vi "LabVIEW Basics #10 - Mouse and Keyboard Control.vi"() -> ()   [LabVIEW 2020]
uses:
  <vilib>/MakerHub/LINX/Public/Utilities/Open Serial.vi
  <vilib>/MakerHub/LINX/Public/Sensors/Motion/Servo/Servo Open N Channels.vi
  <vilib>/MakerHub/LINX/Public/Sensors/Motion/Servo/Servo Set Pulse Width N Channels.vi
  <vilib>/MakerHub/LINX/Public/Sensors/Motion/Servo/Servo Close N Channels.vi
  <vilib>/MakerHub/LINX/LMH-LINX.lvlib
  <vilib>/MakerHub/LINX/Public/Sensors/Motion/Servo/Servo.lvlib
panel:
  out "Mouse Control":picture
  in  "Pan Servo":u16(slide)=2200 step=100 scale=500.0..2500.0
  in  "Tilt Servo":u16(slide)=1400 step=100 scale=500.0..2500.0
  in  "Servo Channels":u8[](array[numeric])
  out "Device Name":string
  in  "Stop":bool
  # "General Controls"
  # "Servo Controls"
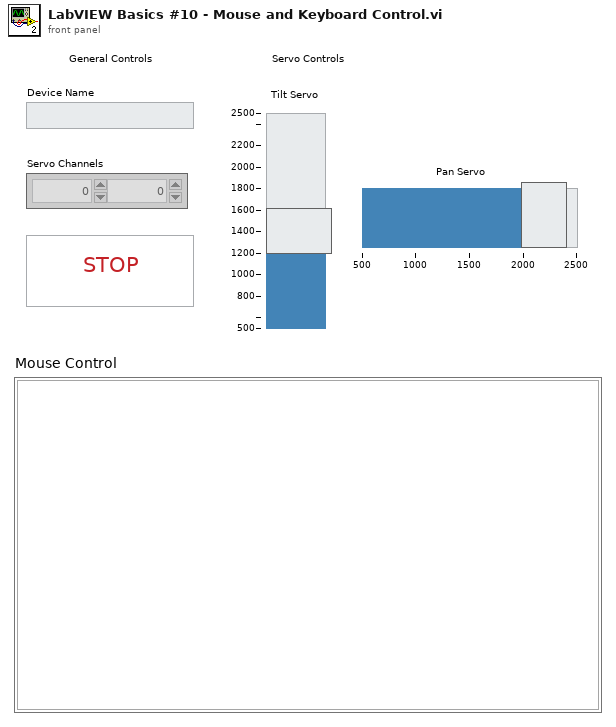
[diagram p1: front panel]
types:
  T1 = typedef "LMH-LINX.lvlib/LINX Ref.ctl" = cluster{"IO":T2, "Interface":T3, "LINX Device Config":T4}
  T2 = typedef "LMH-LINX.lvlib/Platform.ctl" = enum16{"Remote", "Local"}
  T3 = typedef "LMH-LINX.lvlib/Interface.ctl" = enum16{"Serial", "TCP"}
  T4 = typedef "LMH-LINX.lvlib/Device.lvlib/LINX Device Config.ctl" = cluster{"Interface":T3, "COM Port":refnum<visa-resource-name>, "TCP Configuration":T5, "Device Family":u8, "Device ID":u8, "Device Name":string, "TCP Ref":refnum<k5>, "Channels":T6}
  T5 = typedef "LMH-LINX.lvlib/Device.lvlib/TCP Config.ctl" = cluster{"IP Address":string, "Port":u16}
  T6 = typedef "LMH-LINX.lvlib/Channels.ctl" = cluster{"DI":u8[], "DO":u8[], "AI":u8[], "AO":u8[], "PWM":u8[], "QE":u8[], "UART":u8[], "I2C 2":u8[], "SPI":u8[], "CAN":u8[], "Servo":u8[], "AI Ref (V)":dbl, "AI Resolution (Bits)":u8, "AO Ref (V)":dbl, "AO Resolution (Bits)":u8}
  T7 = typedef "eventvkey.ctl" = enum16{"ASCII", "Enter", "Return", "Shift", "Ctrl", "Alt", "Cmd", "Opt", "Caps", "NumLock", "Clear", "Break", "Up", "Down", "Left", "Right", "Insert", "Delete", "Home", "End", "PageUp", "PageDown", "Escape", "Help", "Pause", "ScrollLock", "F1", "F2", "F3", "F4", "F5", "F6", "F7", "F8", "F9", "F10", "F11", "F12", "F13", "F14", "F15", "F16", "F17", "F18", "F19", "F20", "F21", "F22", "F23", "F24", "Play", "VolumeUp", "VolumeDown", "Mute", "Two Byte Char"}
  T8 = typedef "LVMouseTypeDef.ctl" = cluster{"Mouse Position":cluster{"X":i32, "Y":i32}, "Mouse Modifiers":cluster{"Button Down":bool, "Shift Mod":bool, "Menu Mod":bool, "Option Mod":bool}}
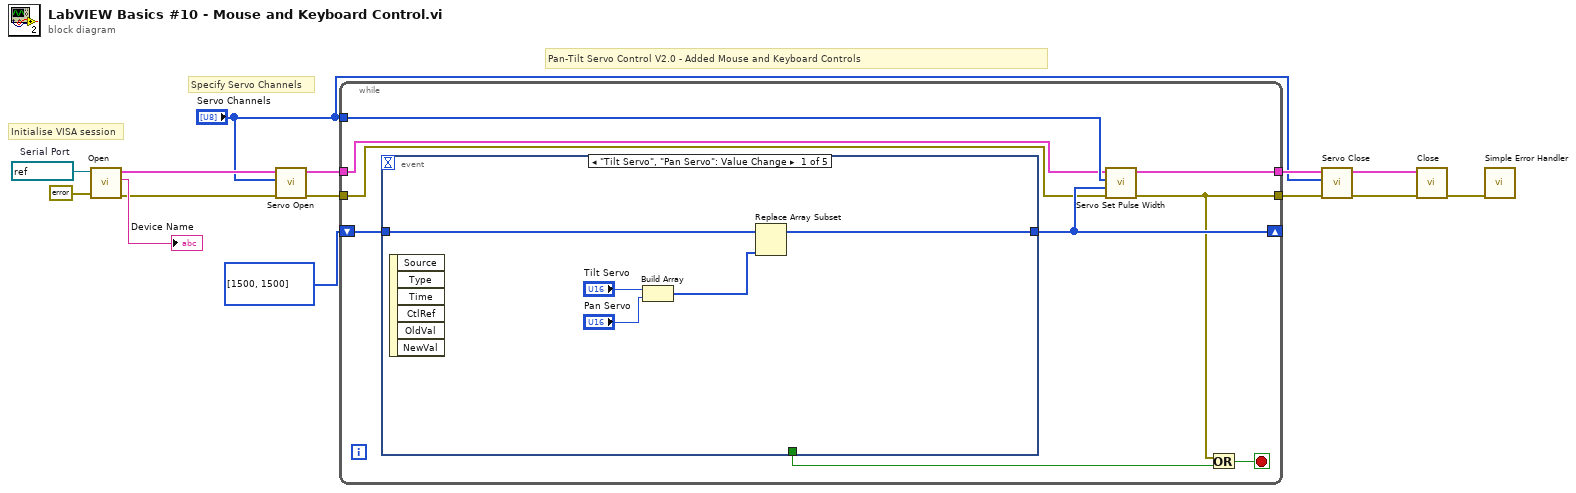
[diagram p0: block diagram]
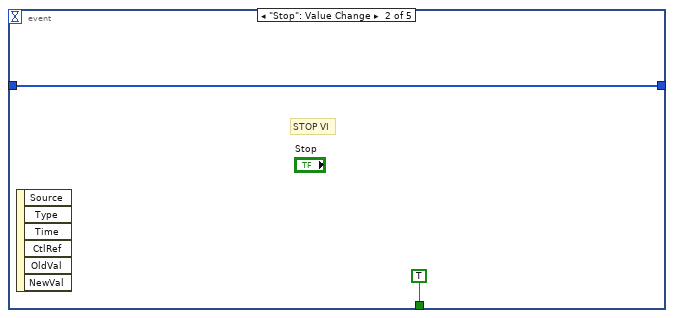
[diagram p2: hidden frame]
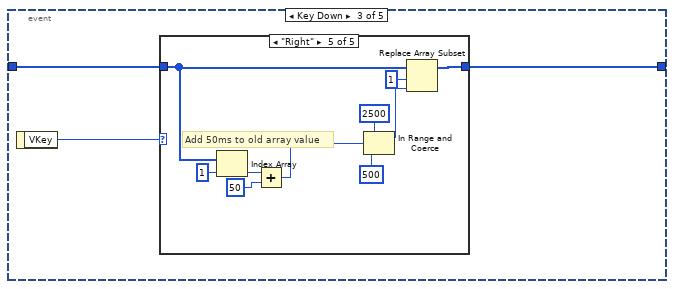
[diagram p3: hidden frame]
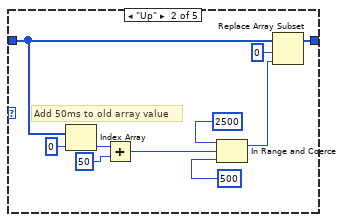
[diagram p5: hidden frame]
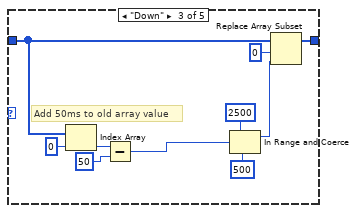
[diagram p6: hidden frame]
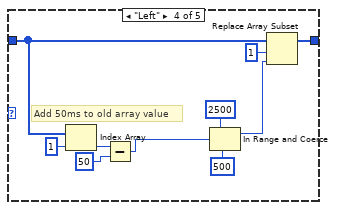
[diagram p7: hidden frame]
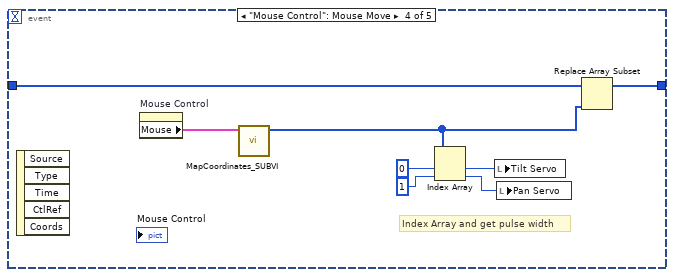
[diagram p8: hidden frame]
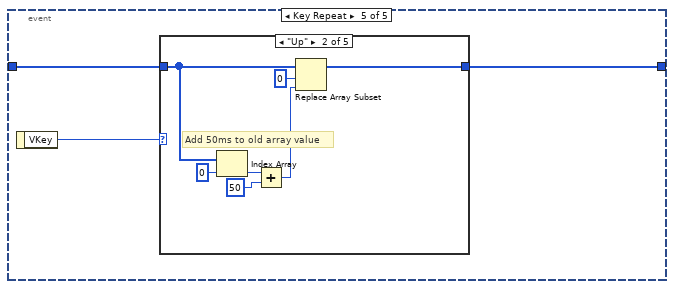
[diagram p9: hidden frame]
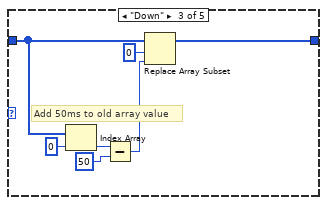
[diagram p11: hidden frame]
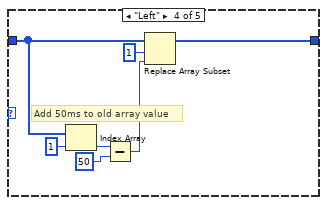
[diagram p12: hidden frame]
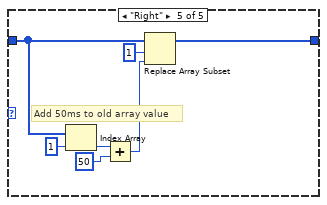
[diagram p13: hidden frame]
diagram:
  w14 = refnum<visa-resource-name> "COM5"  # Serial Port
  # "Specify Servo Channels"
  # "Initialise VISA session"
  # "Pan-Tilt Servo Control V2.0 - Added Mouse and Keyboard Controls"
  n1 = call-poly <vilib>:"Open.vi"("Error In"=errorcluster {"status"=FALSE, "code"=0, "source"=""}, "Serial Port"=w14) -> ("Error Out"=w7:errorcluster, "Device Name"=→"Device Name":string, "LINX Resource"=w6:T1)  [unwired: 7 in]
  n2 = call-poly <vilib>:"Servo Open.vi"("Error In"=w7, "Servo Channels"="Servo Channels", "LINX Resource"=w6) -> ("Error Out"=w5:errorcluster, "LINX Resource"=w8:T1)  [unwired: 7 in]
  n3 = while {
    tunnel: w8 -> [w18]
    tunnel: w5 -> [w17]
    tunnel: "Servo Channels" -> [w20]
    shift-right: [w19] -> _
    shift-left: u16[] [1500, 1500] -> [w21]
    tunnel: [w16] -> w4
    tunnel: [w15] -> w3
    stop <- w23 stop-if-true
    n4 = event shown="[0] \"Tilt Servo\", \"Pan Servo\": Value Change" {
      selector: _ -> [_ _ _ _ _]
      dyn-events: _ -> [_ _ _ _ _]
      timeout: _ -> [_ _ _ _ _]
      tunnel: [_ TRUE ("Stop") _ _ _] -> w22
      tunnel: [w25 w29 w31 w81 w83] -> w19
      tunnel: w21 -> [w26 w29 w32 w80 w84]
      event "Tilt Servo", "Pan Servo": Value Change {
        n5 = event-data() -> ()  [unwired: 1 in, 6 out]
        n6 = Build Array("Tilt Servo", "Pan Servo") -> (w24:u16[])
        n7 = Replace Array Subset(array=w26, new element=w24) -> (w25:u16[])  [unwired: 1 in]
      }
      event "Stop": Value Change {
        # "STOP VI"
        n8 = event-data() -> ()  [unwired: 1 in, 6 out]
      }
      event Key Down {
        n9 = event-data() -> ("VKey"=w33:T7)  [unwired: 1 in]
        n10 = case shown="\"Right\"" w33 {
          tunnel: w32 -> [w34 w42 w52 w62 w72]
          tunnel: [w34 w44 w54 w64 w74] -> w31
          frame "ASCII", Default {
            # "do nothing"
          }
          frame "Up" {
            # "Add 50ms to old array value"
            n11 = Index Array(array=w42, index=0) -> (element=w40:u16)
            n12 = Add(x=w40, y=u16 50) -> (x+y=w38:u16)
            n13 = In Range and Coerce(upper limit=u16 2500, x=w38, lower limit=u16 500 ("x+y")) -> (coerced(x)=w36:u16)  [unwired: 1 out]
            n14 = Replace Array Subset(array=w42, new element=w36, index=0) -> (w44:u16[])
          }
          frame "Down" {
            # "Add 50ms to old array value"
            n15 = Index Array(array=w52, index=0) -> (element=w50:u16)
            n16 = Subtract(x=w50, y=u16 50) -> (x-y=w46:u16)
            n17 = In Range and Coerce(upper limit=u16 2500, x=w46, lower limit=u16 500 ("x+y")) -> (coerced(x)=w45:u16)  [unwired: 1 out]
            n18 = Replace Array Subset(array=w52, new element=w45, index=0) -> (w54:u16[])
          }
          frame "Left" {
            # "Add 50ms to old array value"
            n19 = Index Array(array=w62, index=1) -> (element=w60:u16)
            n20 = Subtract(x=w60, y=u16 50) -> (x-y=w55:u16)
            n21 = In Range and Coerce(upper limit=u16 2500, x=w55, lower limit=u16 500 ("x+y")) -> (coerced(x)=w58:u16)  [unwired: 1 out]
            n22 = Replace Array Subset(array=w62, new element=w58, index=1) -> (w64:u16[])
          }
          frame "Right" {
            # "Add 50ms to old array value"
            n23 = Index Array(array=w72, index=1) -> (element=w70:u16)
            n24 = Add(x=w70, y=u16 50) -> (x+y=w66:u16)
            n25 = In Range and Coerce(upper limit=u16 2500, x=w66, lower limit=u16 500 ("x+y")) -> (coerced(x)=w65:u16)  [unwired: 1 out]
            n26 = Replace Array Subset(array=w72, new element=w65, index=1) -> (w74:u16[])
          }
        }
      }
      event "Mouse Control": Mouse Move {
        # "Index Array and get pulse width"
        n27 = event-data() -> ()  [unwired: 1 in, 5 out]
        n28 = property on="Mouse Control" class="Pict"() -> ("Mouse"=w82:T8)  [unwired: 2 in, 2 out]
        n29 = call "MapCoordinates_SUBVI.vi"("Mouse"=w82) -> ("Pulse Width Array"=w79:u16[])  [unwired: 10 in]
        n30 = Index Array(array=w79, index #1=0 ("index"), index #2=1 ("index")) -> (element #1=w75:u16, element #2=w76:u16)
        n31 = local write "Tilt Servo"(w75) -> ()
        n32 = local write "Pan Servo"(w76) -> ()
        n33 = Replace Array Subset(array=w80, new element=w79) -> (w81:u16[])  [unwired: 1 in]
      }
      event Key Repeat {
        n34 = event-data() -> ("VKey"=w85:T7)  [unwired: 1 in]
        n35 = case shown="\"Up\"" w85 {
          tunnel: w84 -> [w86 w91 w98 w105 w112]
          tunnel: [w86 w93 w100 w107 w114] -> w83
          frame "ASCII", Default {
            # "do nothing"
          }
          frame "Up" {
            # "Add 50ms to old array value"
            n36 = Index Array(array=w91, index=0) -> (element=w89:u16)
            n37 = Add(x=w89, y=u16 50) -> (x+y=w87:u16)
            n38 = Replace Array Subset(array=w91, new element=w87, index=0) -> (w93:u16[])
          }
          frame "Down" {
            # "Add 50ms to old array value"
            n39 = Index Array(array=w98, index=0) -> (element=w96:u16)
            n40 = Subtract(x=w96, y=u16 50) -> (x-y=w94:u16)
            n41 = Replace Array Subset(array=w98, new element=w94, index=0) -> (w100:u16[])
          }
          frame "Left" {
            # "Add 50ms to old array value"
            n42 = Index Array(array=w105, index=1) -> (element=w103:u16)
            n43 = Subtract(x=w103, y=u16 50) -> (x-y=w101:u16)
            n44 = Replace Array Subset(array=w105, new element=w101, index=1) -> (w107:u16[])
          }
          frame "Right" {
            # "Add 50ms to old array value"
            n45 = Index Array(array=w112, index=1) -> (element=w110:u16)
            n46 = Add(x=w110, y=u16 50) -> (x+y=w108:u16)
            n47 = Replace Array Subset(array=w112, new element=w108, index=1) -> (w114:u16[])
          }
        }
      }
    }
    n48 = call-poly <vilib>:"Servo Set Pulse Width.vi"("Error In"=w17, "Pulse Widths (uS)"=w19, "Servo Channels"=w20, "LINX Resource"=w18) -> ("Error Out"=w15:errorcluster, "LINX Resource"=w16:T1)  [unwired: 6 in]
    n49 = Or(x=w15, y=w22) -> (x .or. y?=w23:bool)
  }
  n50 = call-poly <vilib>:"Servo Close.vi"("Error In"=w3, "Servo Channels"="Servo Channels", "LINX Resource"=w4) -> ("Error Out"=w10:errorcluster, "LINX Resource"=w9:T1)  [unwired: 7 in]
  n51 = call <vilib>:"Close.vi"("Error In"=w10, "LINX Resource"=w9) -> ("Error Out"=w11:errorcluster)  [unwired: 9 in]
  n52 = call <vilib>:"Simple Error Handler.vi"("error in (no error)"=w11) -> ()  [unwired: 4 in, 5 out]
